vi "_MainOpenMV.vi"() -> ()   [LabVIEW 2022 SP3]
uses:
  <vilib>/Instr/_visa.llb/VISA Configure Serial Port (Instr).vi
panel:
  in  "VISA resource name":refnum<visa-resource-name>="ASRL30::INSTR"
  in  "stop":bool
  out "new picture":picture
  out "size()":u32[](array[numeric])=[320, 240, 3845, 3100222628, 2249475409, 4188412193, 994418530, 2704393609, 2315364096, 1232119080, 1457127203, 3699463832]
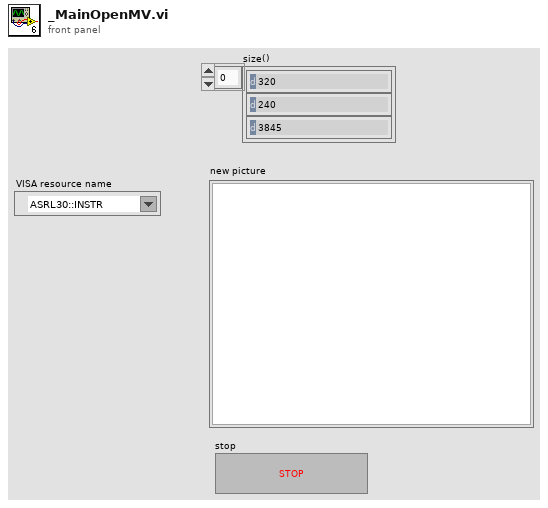
[diagram p1: front panel]
types:
  T1 = typedef "PythonCtrl.ctl" = cluster{"session":refnum<k35>, "PyPath":path, "Processor":T2, "Port":string, "version":string}
  T2 = typedef "Processors.ctl" = enum16{"SPIKE", "Pi", "Pi_ssh", "OpenMV", "Dunio"}
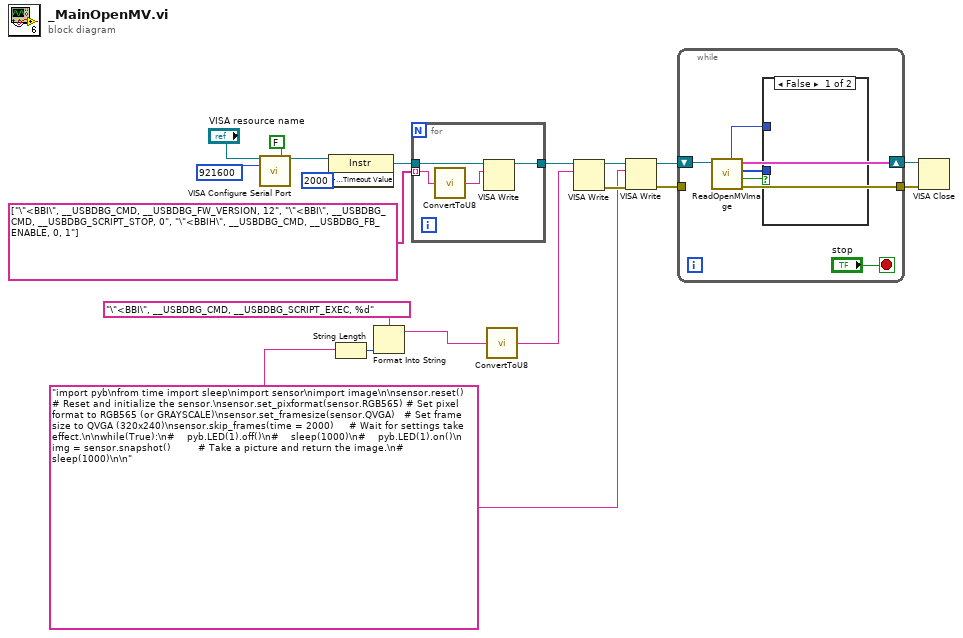
[diagram p0: block diagram]
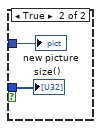
[diagram p2: hidden frame]
diagram:
  w6 = "import pyb\nfrom time import sleep\nimport sensor\nimport image\n\nsensor.reset()                      # Reset and initialize the sensor.\nsensor.set_pixformat(sensor.RGB565) # Set pixel format to RGB565 (or GRAYSCALE)\nsensor.set_framesize(sensor.QVGA)   # Set frame size to QVGA (320x240)\nsensor.skip_frames(time = 2000)     # Wait for settings take effect.\n\nwhile(True):\n#    pyb.LED(1).off()\n#    sleep(1000)\n#    pyb.LED(1).on()\n    img = sensor.snapshot()         # Take a picture and return the image.\n#    sleep(1000)\n\n" ("header buffer")
  # "\"<BBI\", __USBDBG_CMD, __USBDBG_SCRIPT_EXEC, len(buf))"
  n1 = call-poly "VISA Configure Serial Port"("VISA resource name"="VISA resource name", "Enable Termination\nChar (T)"=FALSE ("Enable Termination\nChar (T)"), "baud rate (9600)"=u32 921600 ("baud rate (115200)")) -> ("VISA resource name out"=w3:refnum<visa-resource-name>)  [unwired: 11 in, 1 out]
  n2 = property class="Instr"(reference=w3, "General Settings:Timeout Value"=u32 2000) -> (reference out=w2:refnum<visa-resource-name>)  [unwired: 1 in, 1 out]
  n3 = String Length(string=w6) -> (length=w14:i32)
  n4 = Format Into String(format string="\"<BBI\", __USBDBG_CMD, __USBDBG_SCRIPT_EXEC, %d" ("write buffer"), w14) -> (resulting string=w11:string)  [unwired: 2 in, 1 out]
  n5 = for {
    tunnel: w2 -> [w23]
    tunnel: string[] ["\"<BBI\", __USBDBG_CMD, __USBDBG_FW_VERSION, 12", "\"<BBI\", __USBDBG_CMD, __USBDBG_SCRIPT_STOP, 0", "\"<BBIH\", __USBDBG_CMD, __USBDBG_FB_ENABLE, 0, 1"] -> [w22] mode=indexing
    tunnel: [w20] -> w9
    n6 = call "ConvertToU8.vi"("struct"=w22) -> ("Binary"=w21:string)
    n7 = VISA Write(VISA resource name=w23, write buffer=w21) -> (VISA resource name out=w20:refnum<visa-resource-name>)  [unwired: 1 in, 2 out]
  }
  n8 = call "ConvertToU8.vi"("struct"=w11) -> ("Binary"=w10:string)
  n9 = VISA Write(VISA resource name=w9, write buffer=w10) -> (VISA resource name out=w7:refnum<visa-resource-name>, error out=w8:errorcluster)  [unwired: 1 in, 1 out]
  n10 = VISA Write(VISA resource name=w7, write buffer=w6, error in (no error)=w8) -> (VISA resource name out=w1:refnum<visa-resource-name>, error out=w5:errorcluster)  [unwired: 1 out]
  n11 = while {
    tunnel: [w29] -> w16
    shift-right: [w28] -> w15
    shift-left: w1 -> [w30]
    tunnel: w5 -> [_]
    stop <- "stop" stop-if-true
    n12 = call "ReadOpenMVImage.vi"("Python"=w30) -> ("error out"=w29:errorcluster, "Good?"=w24:bool, "size()"=w26:u32[], "Python"=w28:T1, "new picture"=w27:picture)  [unwired: 5 in, 1 out]
    n13 = case shown="False" w24 {
      tunnel: w27 -> [_ w32]
      tunnel: w26 -> [_ w31]
      frame False {
      }
      frame True {
        "size()" <- w31
        "new picture" <- w32
      }
    }
  }
  n14 = VISA Close(VISA resource name=w15, error in (no error)=w16) -> ()  [unwired: 1 out]
